vi "FTW-JSON-Construct-FromPointer.vi"(5 "JSON Object Pointer":i64, 11 "error in":errorcluster) -> (4 "JSON Object":T1, 15 "error out":errorcluster)   [LabVIEW 2015, in "FTW-JSON.lvclass"]
uses:
  FTW-JSON.lvclass
  core/type/FTW-Type-JSON.ctl
panel:
  # "Inputs"
  # "Outputs"
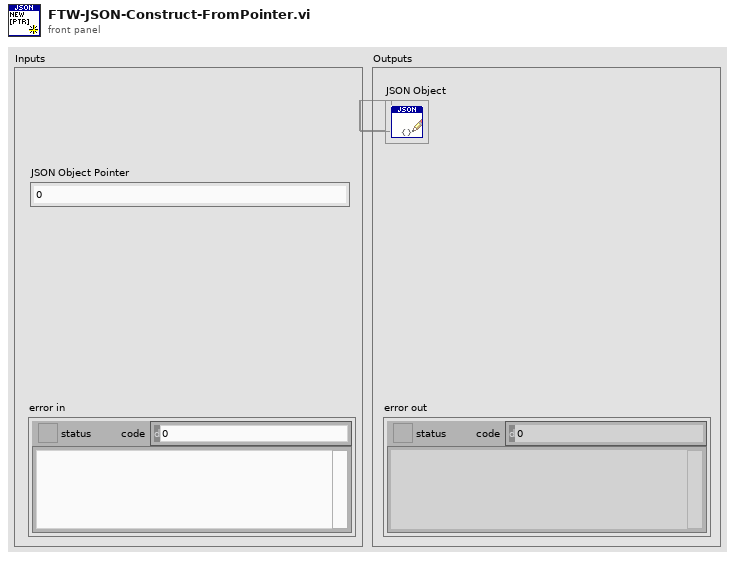
[diagram p1: front panel]
types:
  T1 = typedef "FTW-Type-JSON.ctl" = refnum<data-value>
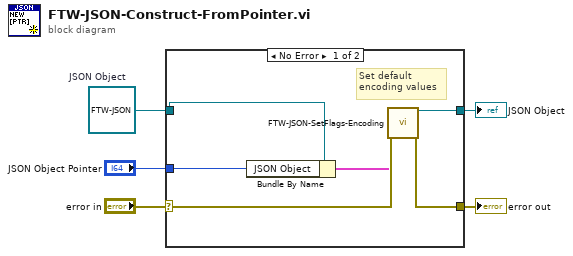
[diagram p0: block diagram]
diagram:
  w4 = refnum<class "FTW-JSON.lvclass"> refnum  # JSON Object
  n1 = case shown="No Error" "error in" {
    selector: "error in" -> [w10 w13]
    tunnel: [w6 w13] -> w5
    tunnel: [w7 w12] -> w3
    tunnel: w4 -> [w11 w12]
    tunnel: "JSON Object Pointer" -> [w9 _]
    frame No Error {
      # "Set default\nencoding values"
      n2 = Bundle By Name(cluster=w11, "JSON Object"=w9) -> (w8:cluster{})
      n3 = call "FTW-JSON-SetFlags-Encoding.vi"("JSON Object"=w8, "error in"=w10) -> ("JSON Object out"=w7:refnum<class "FTW-JSON.lvclass">, "error out"=w6:errorcluster)  [unwired: 12 in]
    }
    frame Error {
    }
  }
  "error out" <- w5
  "JSON Object" <- w3
